vi "Cut_Unmoving_Dots_from_(X,Y)-1.vi"(0 "[IN] (X,Y)":dbl[][](array[numeric]), 1 "Gap closed!!!":bool, 2 "Index of \ncandidate dot\ninside the frame":i32, 5 "Count of gaps \nbetween dots":i32, 7 "i+j":i32, 9 "[IN] Array for collecting \nunmoving dots tree":dbl[](array[numeric]), 11 "Starting\nIndex for\nUnmov Tree":i32, 12 "previous dot\nindex in column":i32, 13 "previous \ndot # frame":i32) -> (4 "[OUT] (X,Y)":dbl[][](array[numeric]), 10 "[OUT] Array for collecting \nunmoving dots tree":dbl[](array[numeric]), 15 "Finish\nIndex":i32)   [LabVIEW 2013]
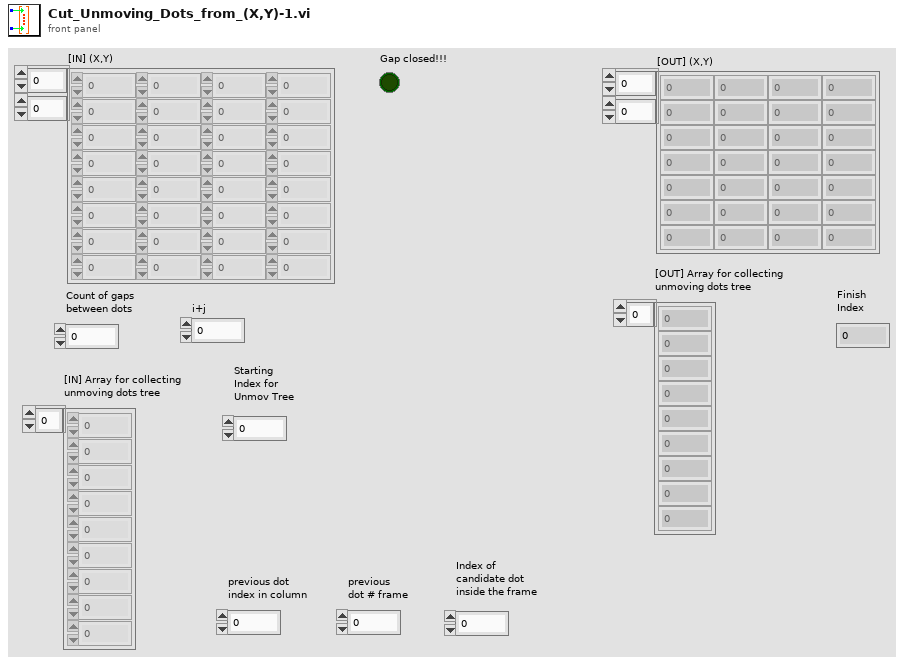
[diagram p1: front panel]
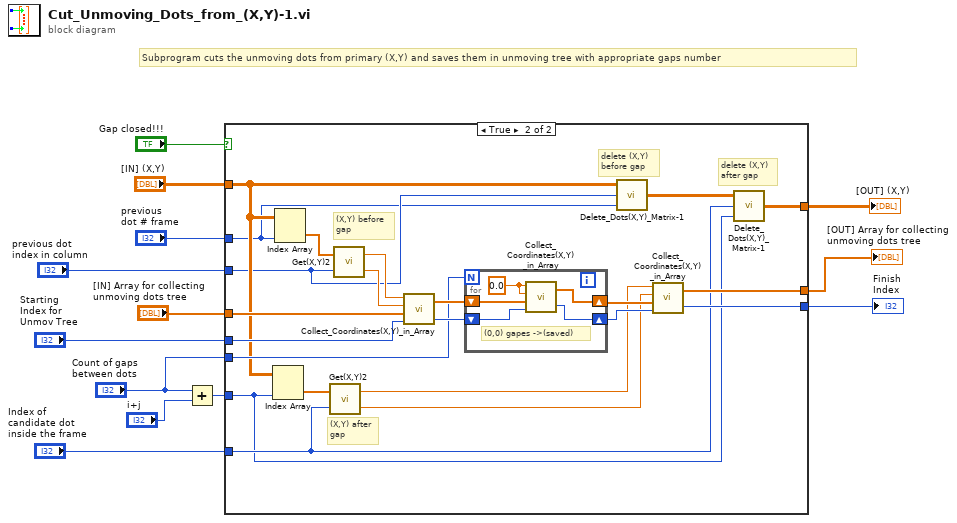
[diagram p0: block diagram]
diagram:
  # "Subprogram cuts the unmoving dots from primary (X,Y) and saves them in unmoving tree with appropriate gaps number"
  n1 = Add(x="Count of gaps \nbetween dots", y="i+j") -> (x+y=w5:i32)
  n2 = case shown="True" "Gap closed!!!" {
    tunnel: "[IN] (X,Y)" -> [w16 w29]
    tunnel: "previous \ndot # frame" -> [_ w21]
    tunnel: "previous dot\nindex in column" -> [_ w22]
    tunnel: "[IN] Array for collecting \nunmoving dots tree" -> [w15 w35]
    tunnel: "Starting\nIndex for\nUnmov Tree" -> [w14 w34]
    tunnel: "Index of \ncandidate dot\ninside the frame" -> [_ w18]
    tunnel: w5 -> [_ w17]
    tunnel: "Count of gaps \nbetween dots" -> [_ w31]
    tunnel: [w15 w24] -> w2
    tunnel: [w14 w23] -> w3
    tunnel: [w16 w19] -> w1
    frame False {
    }
    frame True {
      # "delete (X,Y)\nafter gap"
      # "delete (X,Y)\nbefore gap"
      # "(X,Y) after\ngap"
      # "(X,Y) before\ngap"
      n3 = Index Array(array=w29, index (col)=w17) -> (element=w30:dbl[])  [unwired: 1 in]
      n4 = Index Array(array=w29, index (col)=w21) -> (element=w38:dbl[])  [unwired: 1 in]
      n5 = call "Get(X,Y)2.vi"("[IN] index of (X,Y)"=w18, "[IN] Array coordi\nnates (X,Y) in Frame"=w30) -> ("[OUT] Y"=w25:dbl, "[OUT] X"=w26:dbl)
      n6 = call "Get(X,Y)2.vi"("[IN] index of (X,Y)"=w22, "[IN] Array coordi\nnates (X,Y) in Frame"=w38) -> ("[OUT] Y"=w36:dbl, "[OUT] X"=w37:dbl)
      n7 = call "Collect_Coordinates(X,Y)_in_Array.vi"("Initial Index \nfor Replacement"=w34, "[IN] Array for \nCollecting \nCoord (X,Y)"=w35, "Y"=w36, "X"=w37) -> ("Finish\nIndex"=w32:i32, "[OUT] Array\nfor collecting"=w33:dbl[])
      n8 = for {
        N: w31 -> [_]
        shift-right: [w40] -> w28
        shift-left: w33 -> [w42]
        shift-right: [w39] -> w27
        shift-left: w32 -> [w43]
        w41 = 0.0 ("X")
        # "(0,0) gapes ->(saved)"
        n9 = call "Collect_Coordinates(X,Y)_in_Array.vi"("Initial Index \nfor Replacement"=w43, "[IN] Array for \nCollecting \nCoord (X,Y)"=w42, "Y"=w41, "X"=w41) -> ("Finish\nIndex"=w39:i32, "[OUT] Array\nfor collecting"=w40:dbl[])
      }
      n10 = call "Delete_Dots(X,Y)_Matrix-1.vi"("# Frame"=w21, "# Dot"=w22, "(X,Y) IN"=w29) -> ("(X,Y) OUT"=w20:dbl[][])
      n11 = call "Collect_Coordinates(X,Y)_in_Array.vi"("Initial Index \nfor Replacement"=w27, "[IN] Array for \nCollecting \nCoord (X,Y)"=w28, "Y"=w25, "X"=w26) -> ("Finish\nIndex"=w23:i32, "[OUT] Array\nfor collecting"=w24:dbl[])
      n12 = call "Delete_Dots(X,Y)_Matrix-1.vi"("# Frame"=w17, "# Dot"=w18, "(X,Y) IN"=w20) -> ("(X,Y) OUT"=w19:dbl[][])
    }
  }
  "Finish\nIndex" <- w3
  "[OUT] Array for collecting \nunmoving dots tree" <- w2
  "[OUT] (X,Y)" <- w1
